vi "Log File.vi"(5 "Y direction steps":i32, 7 "X direction steps":i32, 8 "Step size":i32, 9 "User input notes (ENTER)":string, 10 "operation (0:open)":T1(ring)) -> (0 "error out":errorcluster, 3 "path":path)   [LabVIEW 2015]
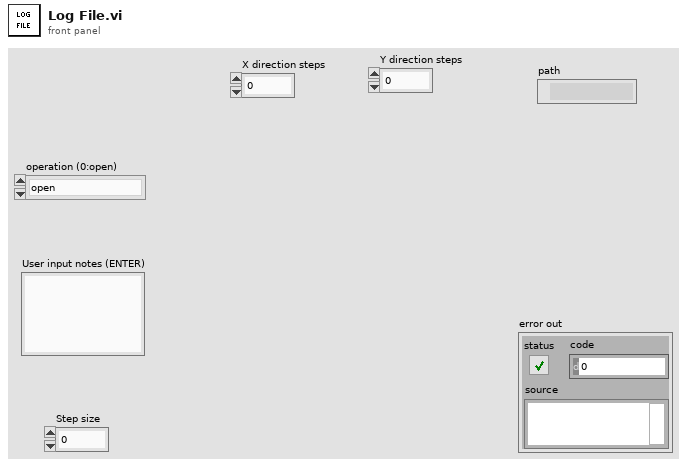
[diagram p1: front panel]
types:
  T1 = enum16{"open", "replace", "create", "open or create", "replace or create", "replace or create with confirmation"}
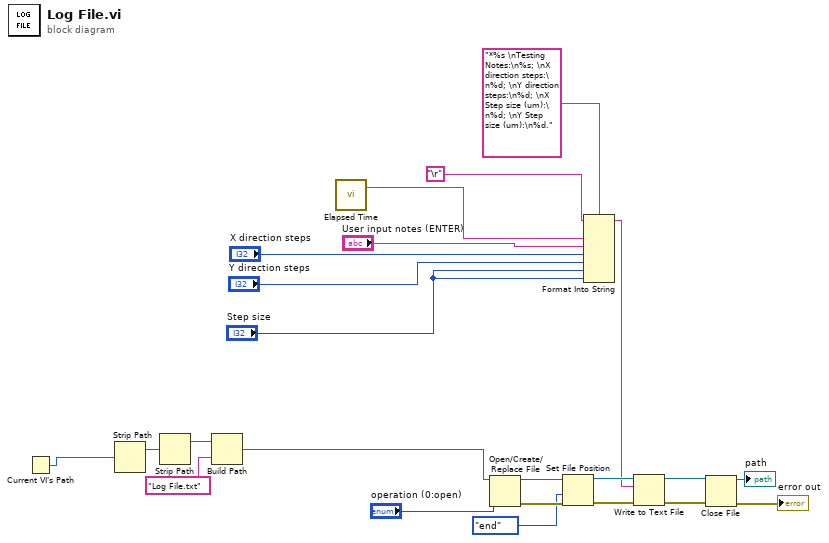
[diagram p0: block diagram]
diagram:
  n1 = Current VI's Path() -> (path=w1:path)
  n2 = Strip Path(path=w1) -> (stripped path=w5:path)  [unwired: 1 out]
  n3 = Strip Path(path=w5) -> (stripped path=w4:path)  [unwired: 1 out]
  n4 = Build Path(base path=w4, name or relative path="Log File.txt") -> (appended path=w2:path)
  n5 = call "Elapsed Time"() -> ("Present Text"=w14:string)  [unwired: 12 in, 7 out]
  n6 = Open/Create/Replace File(file path (use dialog)=w2, operation (0:open)="operation (0:open)") -> (refnum out=w23:refnum<file>, error out=w22:errorcluster)  [unwired: 4 in, 1 out]
  n7 = Set File Position(refnum=w23, from (0:start)=enum16{"start", "end", "current"}."end", error in=w22) -> (refnum out=w20:refnum<file>, error out=w19:errorcluster)  [unwired: 1 in]
  n8 = Format Into String(format string="*%s \nTesting Notes:\n%s; \nX direction steps:\n%d; \nY direction steps:\n%d; \nX Step size (um):\n%d; \nY Step size (um):\n%d." ("格式字符串"), initial string="\r", w14, "User input notes (ENTER)", "X direction steps", "Y direction steps", "Step size", "Step size") -> (resulting string=w12:string)  [unwired: 1 in, 1 out]
  n9 = Write to Text File(file (use dialog)=w20, text=w12, error in=w19) -> (refnum out=w18:refnum<file>, error out=w17:errorcluster)  [unwired: 1 in, 1 out]
  n10 = Close File(refnum=w18, error in=w17) -> (path=→"path":path, error out=→"error out":errorcluster)
